vi "test launch clientr.vi"() -> ()   [LabVIEW 2016, in "client.lvlib" / "client.lvclass"]
uses:
  client/client/client.lvclass
  C:/Program Files/National Instruments/LabVIEW 2016/vi.lib/ActorFramework/Actor/Actor.lvclass
  <vilib>/ActorFramework/Message Enqueuer/Message Enqueuer.lvclass/Message Enqueuer.ctl
  server Messages/send message to server Msg/send message to server Msg.lvclass/send message to server Msg.ctl
  <vilib>/ActorFramework/Message Enqueuer/Enqueue.vi
  <vilib>/ActorFramework/Stop Msg/Stop Msg.lvclass
  C:/Program Files/National Instruments/LabVIEW 2016/vi.lib/ActorFramework/Message/Message.lvclass
  server Messages/send message to server Msg/send message to server Msg.lvclass
  <vilib>/ActorFramework/Message Priority Queue/Priority Enqueue.vi
  <vilib>/ActorFramework/Message Enqueuer/Message Enqueuer.lvclass
  <vilib>/ActorFramework/Actor/Actor.lvclass
panel:
  in  "event message":string
  in  "send message":bool=TRUE
  in  "stop":bool=TRUE
  # "Launch client"
  # "#这是一个测试client的vi，测试启动、停止server，测试给server发送消息；"
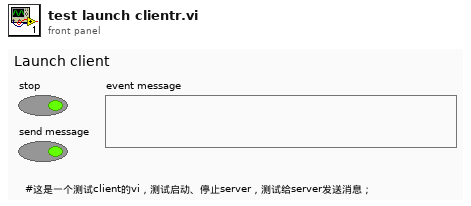
[diagram p1: front panel]
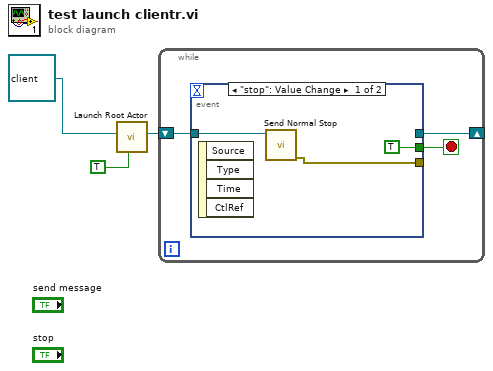
[diagram p0: block diagram]
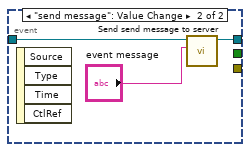
[diagram p2: hidden frame]
diagram:
  n1 = call <vilib>:"Launch Root Actor.vi"("Open Actor Core front panel? (F)"=TRUE, "Actor"=refnum<class "client.lvclass"> refnum ("client.lvlib:client.lvclass")) -> ("Actor's Enqueuer"=w2:refnum<class "Message Enqueuer.lvclass">)  [unwired: 8 in, 1 out]
  n2 = while {
    shift-right: [w4] -> _
    shift-left: w2 -> [w6]
    stop <- w5 stop-if-true
    n3 = event shown="[0] \"stop\": Value Change" {
      selector: _ -> [_ _]
      dyn-events: _ -> [_ _]
      timeout: _ -> [_ _]
      tunnel: w6 -> [w9 w12]
      tunnel: [TRUE _] -> w5
      tunnel: [_ w11] -> w4
      tunnel: [w7 _] -> _
      event "stop": Value Change {
        n4 = event-data() -> ()  [unwired: 1 in, 4 out]
        n5 = call <vilib>:"Send Normal Stop.vi"("Message Enqueuer"=w9) -> ("error out"=w7:errorcluster)  [unwired: 10 in]
      }
      event "send message": Value Change {
        n6 = event-data() -> ()  [unwired: 1 in, 4 out]
        n7 = call "Send send message to server.vi"("event message"="event message", "Message Enqueuer"=w12) -> ("Message Enqueuer out"=w11:refnum<class "Message Enqueuer.lvclass">)  [unwired: 8 in, 1 out]
      }
    }
  }
